vi "Created Remove.vi"(10 "Created Alias":string, 11 "Base Addresses Strategy in":refnum<class "Base Addresses Strategy.lvclass">) -> (3 "Base Addresses Strategy out":refnum<class "Base Addresses Strategy.lvclass">)   [LabVIEW 2021, in "jettl.lvlib" / "Addresses Strategy.lvlib" / "Base Addresses Strategy.lvclass"]
uses:
  Base Addresses Strategy.lvclass
  Base Addresses Strategy.lvclass/Base Addresses Strategy.ctl
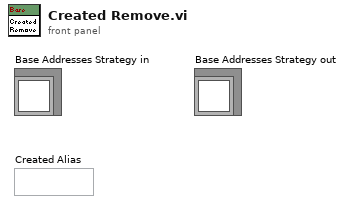
[diagram p1: front panel]
types:
  T1 = typedef "jettl.lvlib/Addresses Strategy.lvlib/Created.ctl" = map{string, refnum<user-event>}
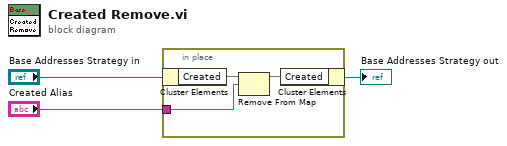
[diagram p0: block diagram]
diagram:
  n1 = in-place {
    in-place-border: "Created Alias" -> [w6]
    n2 = in-place-cluster #1("Base Addresses Strategy in") -> ("Created"=w5:T1)
    n3 = Remove From Map(10:w6, 11:w5) -> (3:w4:T1)  [unwired: 2 out]
    n4 = in-place-cluster #1("Created"=w4) -> (→"Base Addresses Strategy out":refnum<class "Base Addresses Strategy.lvclass">)
  }
